vi "Last Ack Creator Queue.vi"(10 "Queue":refnum<class "Queue.lvclass">, 11 "Last Ack Creator Queue in":refnum<class "Last Ack Creator Queue.lvclass">) -> (3 "Last Ack Creator Queue out":refnum<class "Last Ack Creator Queue.lvclass">)   [LabVIEW 2021, in "jettl.lvlib" / "Last Ack Creator Queue Msg Strategy.lvlib" / "Last Ack Creator Queue.lvclass"]
uses:
  Last Ack Creator Queue.lvclass
  Queue/Queue.lvclass
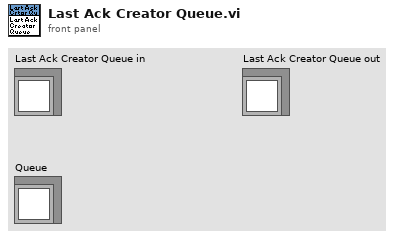
[diagram p1: front panel]
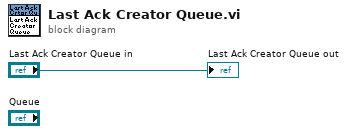
[diagram p0: block diagram]
diagram:
  "Last Ack Creator Queue out" <- "Last Ack Creator Queue in"
